vi "ReadObjectLayout.vi"(7 "properties to ignore":variant, 8 "error in (no error)":errorcluster, 10 "GObj Refnum":refnum<vi>, 11 "Slide Control Layout in":refnum<class "Slide Control Layout.lvclass">) -> (0 "error out":errorcluster, 3 "Slide Control Layout out":refnum<class "Slide Control Layout.lvclass">)   [LabVIEW 2010, in "NI_SE_Front Panel Layout.lvlib" / "Slide Control Layout.lvclass"]
doc: "Read layout information from the GObj Refnum."
uses:
  Slide Control Layout.lvclass
  NumericWithScale Control Layout/NumericWithScale Control Layout.lvclass
  Slide Control Layout.lvclass/Slide Control Layout.ctl
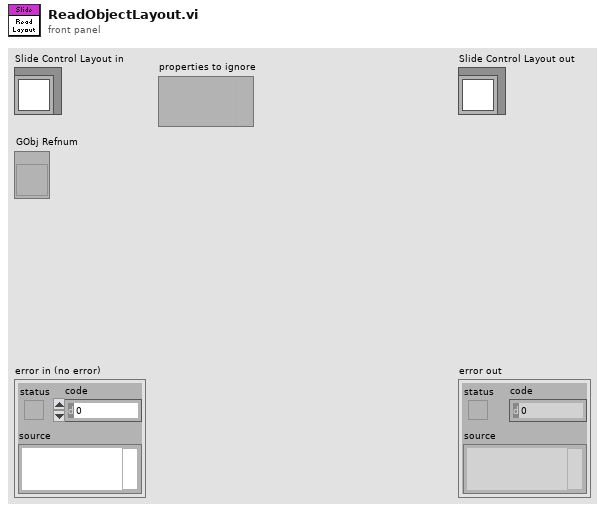
[diagram p1: front panel]
types:
  T1 = typedef "LVFontTypeDef.ctl" = cluster{"Font Name":string, "Size":u16, "Bold":bool, "Italic":bool, "Underline":bool, "Strikeout":bool, "Color":u32}
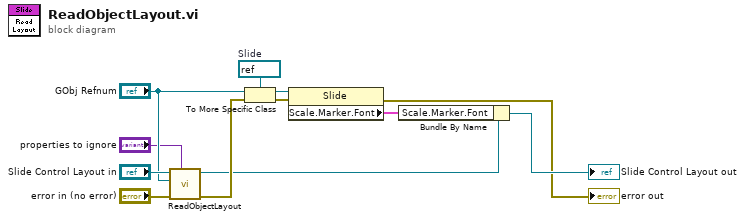
[diagram p0: block diagram]
diagram:
  w4 = refnum<vi> refnum  # Slide
  n1 = call-parent "ReadObjectLayout.vi"("properties to ignore"="properties to ignore", "error in (no error)"="error in (no error)", "GObj Refnum"="GObj Refnum", "NumericWithScale Control Layout in"="Slide Control Layout in") -> ("error out"=w10:errorcluster, "NumericWithScale Control Layout out"=w9:refnum<class "Slide Control Layout.lvclass">)  [unwired: 6 in]
  n2 = To More Specific Class(target class=w4, reference="GObj Refnum", error in=w10) -> (specific class reference=w3:refnum<vi>, error out=w2:errorcluster)
  n3 = property class="Slide"(reference=w3, error in=w2) -> (error out=→"error out":errorcluster, "Scale.Marker.Font"=w1:T1)  [unwired: 1 out]
  n4 = Bundle By Name(cluster=w9, "Scale.Marker.Font"=w1) -> (→"Slide Control Layout out":refnum<class "Slide Control Layout.lvclass">)
